vi "MeasureLockIn.vi"(4 "#Measurements each Frequency":i32=200, 6 "error in":errorcluster, 8 "Stop":dbl=200.0 format="%.2f", 9 "Wait (ms)":dbl=200.0 format="%.2f", 10 "Step":dbl=200.0 format="%.2f", 11 "Start":dbl=200.0 format="%.2f") -> (0 "error out":errorcluster)   [LabVIEW 2010]
panel:
  in  "Path":path
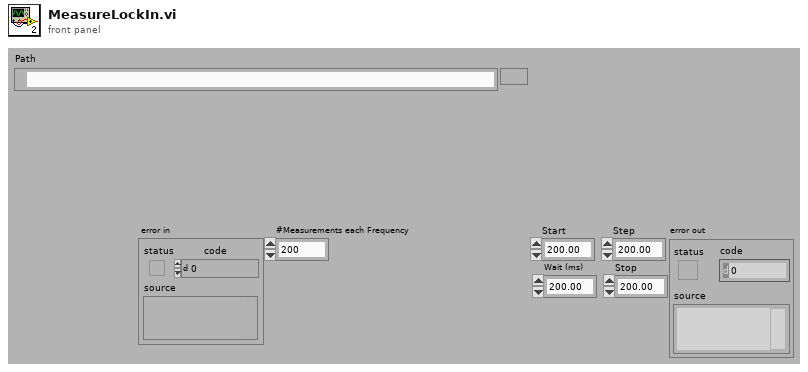
[diagram p1: front panel]
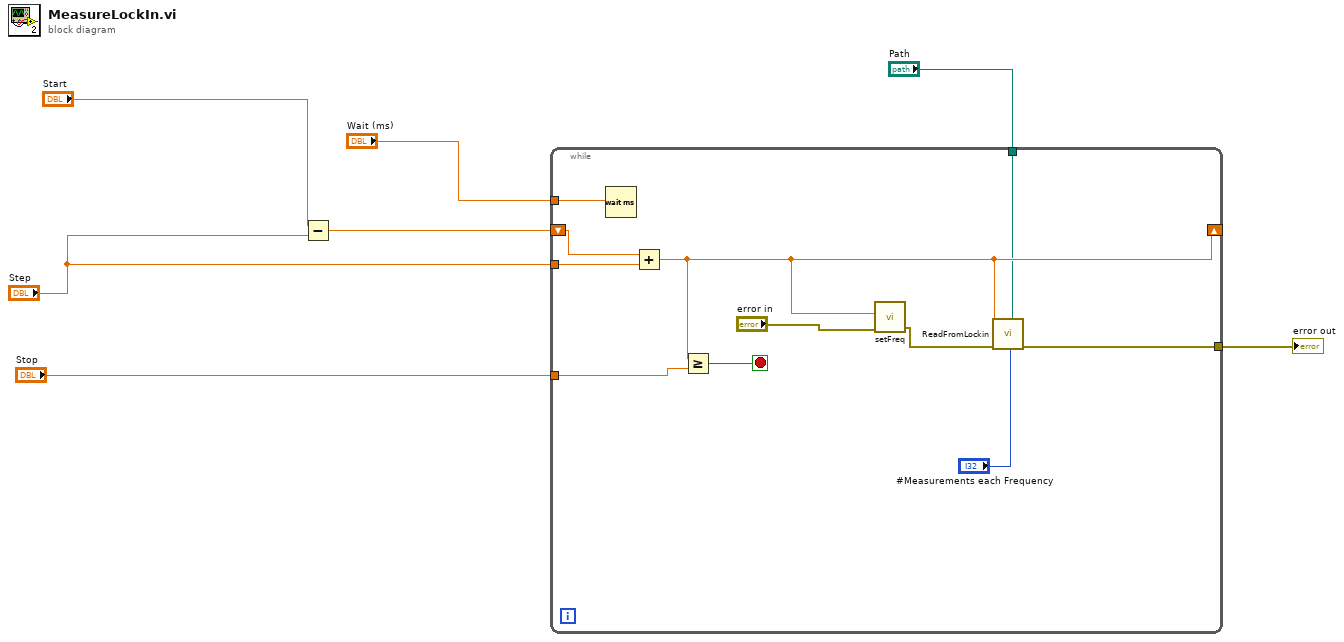
[diagram p0: block diagram]
diagram:
  n1 = Subtract(x="Start", y="Step") -> (x-y=w5:dbl)
  n2 = while {
    tunnel: "Wait (ms)" -> [w14]
    shift-right: [w12] -> _
    shift-left: w5 -> [w18]
    tunnel: "Step" -> [w17]
    tunnel: "Stop" -> [w16]
    tunnel: [w10] -> w2
    tunnel: "Path" -> [w8]
    stop <- w15 stop-if-true
    n3 = Wait (ms)(milliseconds to wait=w14) -> ()  [unwired: 1 out]
    n4 = Add(x=w18, y=w17) -> (x+y=w12:dbl)
    n5 = Greater Or Equal?(x=w12, y=w16) -> (x >= y?=w15:bool)
    n6 = call "setFreq.vi"("error in"="error in", "Frequenz in Hz"=w12) -> ("error out"=w9:errorcluster)  [unwired: 4 in]
    n7 = call "ReadFromLockin.vi"("#Measurements each Frequency"="#Measurements each Frequency", "Path"=w8, "Frequency"=w12, "error in 2"=w9) -> ("error out 2"=w10:errorcluster)  [unwired: 7 in]
  }
  "error out" <- w2
